vi "FXP NILIA_Demodulator.vi"(9 "New Data":bool, 10 "ref":fxp<+/-,24,2>, 11 "signal":fxp<+/-,24,1>) -> (1 "Data Ready":bool, 3 "x*y":i32)   [LabVIEW 2012]
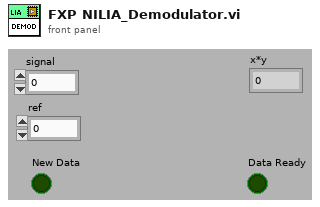
[diagram p1: front panel]
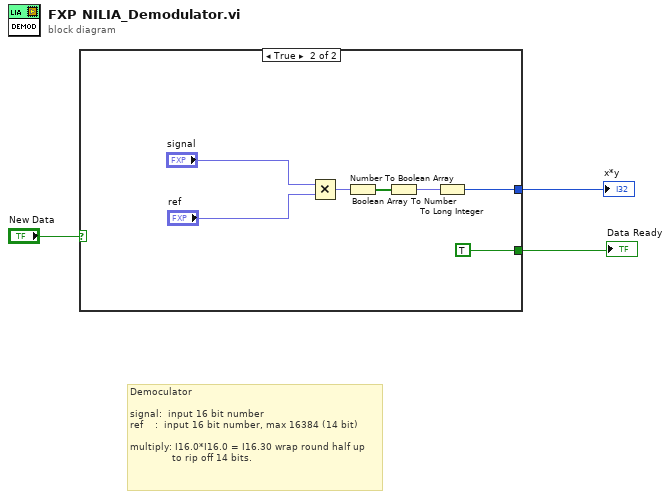
[diagram p0: block diagram]
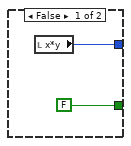
[diagram p2: hidden frame]
diagram:
  # "Democulator\n\nsignal:  input 16 bit number \nref    :  input 16 bit number, max 16384 (14 bit)\n\nmultiply: I16.0*I16.0 = I16.30 wrap round half up\n              to rip off 14 bits."
  n1 = case shown="True" "New Data" {
    tunnel: [w5 w6] -> w2
    tunnel: [FALSE TRUE] -> w1
    frame False {
      n2 = local read "x*y"() -> (w5:i32)
    }
    frame True {
      n3 = Multiply(x="signal", y="ref") -> (x*y=w12:fxp<+/-,24,1>)
      n4 = Number To Boolean Array(number=w12) -> (Boolean array=w11:bool[])
      n5 = Boolean Array To Number(Boolean array=w11) -> (number=w7:fxp<+/-,24,24>)
      n6 = To Long Integer(number=w7) -> (32bit integer=w6:i32)
    }
  }
  "Data Ready" <- w1
  "x*y" <- w2
